vi "Data_Aquisition_cRIO7.vi"() -> ()   [LabVIEW 2016]
uses:
  <vilib>/Platform/TimedLoop/XDataNode/timing_clust.ctl
  <vilib>/Platform/TimedLoop/XDataNode/nitl_modes.ctl
  <vilib>/Platform/TimedLoop/XDataNode/wakeup.ctl
  <vilib>/Utility/file.llb/Write Delimited Spreadsheet (string).vi
  <vilib>/Platform/TimedLoop/XDataNode/loadnilvce.vi
  <vilib>/Utility/file.llb/Write Delimited Spreadsheet (DBL).vi
  <vilib>/Platform/TimedLoop/XDataNode/XDataNode.xnode
  <vilib>/Platform/TimedLoop/XDataNode/XDNodeRunTimeDep.lvlib
panel:
  in  "Mod 8 Labels":string[][](array[string])
  in  "Mod 6 Labels":string[][](array[string])
  in  "Mod 3 Labels":string[][](array[string])
  in  "Mod 2 Labels":string[][](array[string])
  in  "Mod 1 Labels":string[][](array[string])
  out "File Headers":string[][](array[string])=[["Unix Time Code", "M1AI0", "M1AI1", "M1AI2", "M1AI3", "M1AI4", "M1AI5", "M1AI6", "M1AI7", "M2DO0", "M2DO1", "M2DO3  ", "M2DO4", "M2DO4", "M2DO5", "M2DO6", "M2DO7", "M3AO0", "M3AO1", "M3AO2", "M3AO3", "M4DO0", "M4DO1", "M4DO2", "M4DO3", "M4DO4", "M4DO5", "M4DO6", "M4DO7", "M5AI0", "M5AI1", "M5AI2", "M5AI3", "M5AI4", "M5AI5", "M5AI6", "M5AI7", "M6AI0", "M6AI1", "M6AI2", "M6AI3", "M6AI4", "M6AI5", "M6AI6", "M6AI7", "M6AI16", "M6AI7", "M6AI18", "M6AI19", "M6AI20", "M6AI21", "M6AI22", "M6AI23", "M7DO0", "M7DO1", "M7DO3  ", "M7DO4", "M7DO4", "M7DO5", "M7DO6", "M7DO7", "M3AO0", "M3AO1", "M3AO2", "M3AO3"], ["Unix Time Code", "R1 pH", "N/A", "R1 N2  ", "N/A", "R1 Air", "R2 DO", "R2 Air", "R2 N2", "R1 Media Pump", "R1 Water Pump", "R1 Eff Pump", "R1 Gas Pump", "R1 Acid Pump", "R1 Base Pump", "R2 Air Valve", "R1 Release Valve", "R1 Air MFC", "R1 N2 MFC", "N/A", "N/A", "R2 Water Pump", "R2 Media Pump", "R2 Eff Pump", "R2 Acid Pump", "R2 Base Pump", "R2 Gas Pump", "R2 Release Valve", "R2 N2 Valve", "R2 pH", "N/A", "N/A", "N/A", "N/A", "N/A", "N/A", "N/A", "R1 DO ", "N/A", "R1 NH4+", "N/A", "R1 Ca2+", "N/A", "R1 K+", "N/A", "R1 Na+", "N/A", "R1 Cl-", "N/A", "R1 NO3-", "N/A", "R1 ORP", "N/A", "N/A", "N/A", "N/A", "R2 Water Pump 2", "R2 Floc FAir Valve", "R2 Floc Eff Pump", "R2 Floc Return Pump", "N/A", "R1 Air MFC", "R1 N2 MFC", "N/A", "N/A"]]
  in  "Buffer Size":i32=100
  out "Saving?":bool=TRUE
  out "new file path (Not A Path if cancelled)":path=path "u:/_03162018_194505.csv"
  in  "File Name:":string
  out "error out":errorcluster={"status"=TRUE, "code"=7, "source"="Open/Create/Replace File in Write Spreadsheet String.vi->Write Delimited Spreadsheet (string).vi->Data_Aquisition_cRIO1.vi<APPEND>\n/u/_03132018_011937.csv"}
  out "iter number":i32=109873
  in  "stop":bool
  out "All data":dbl[][](array[numeric]) format="%#3.4f"
  in  "error in":errorcluster
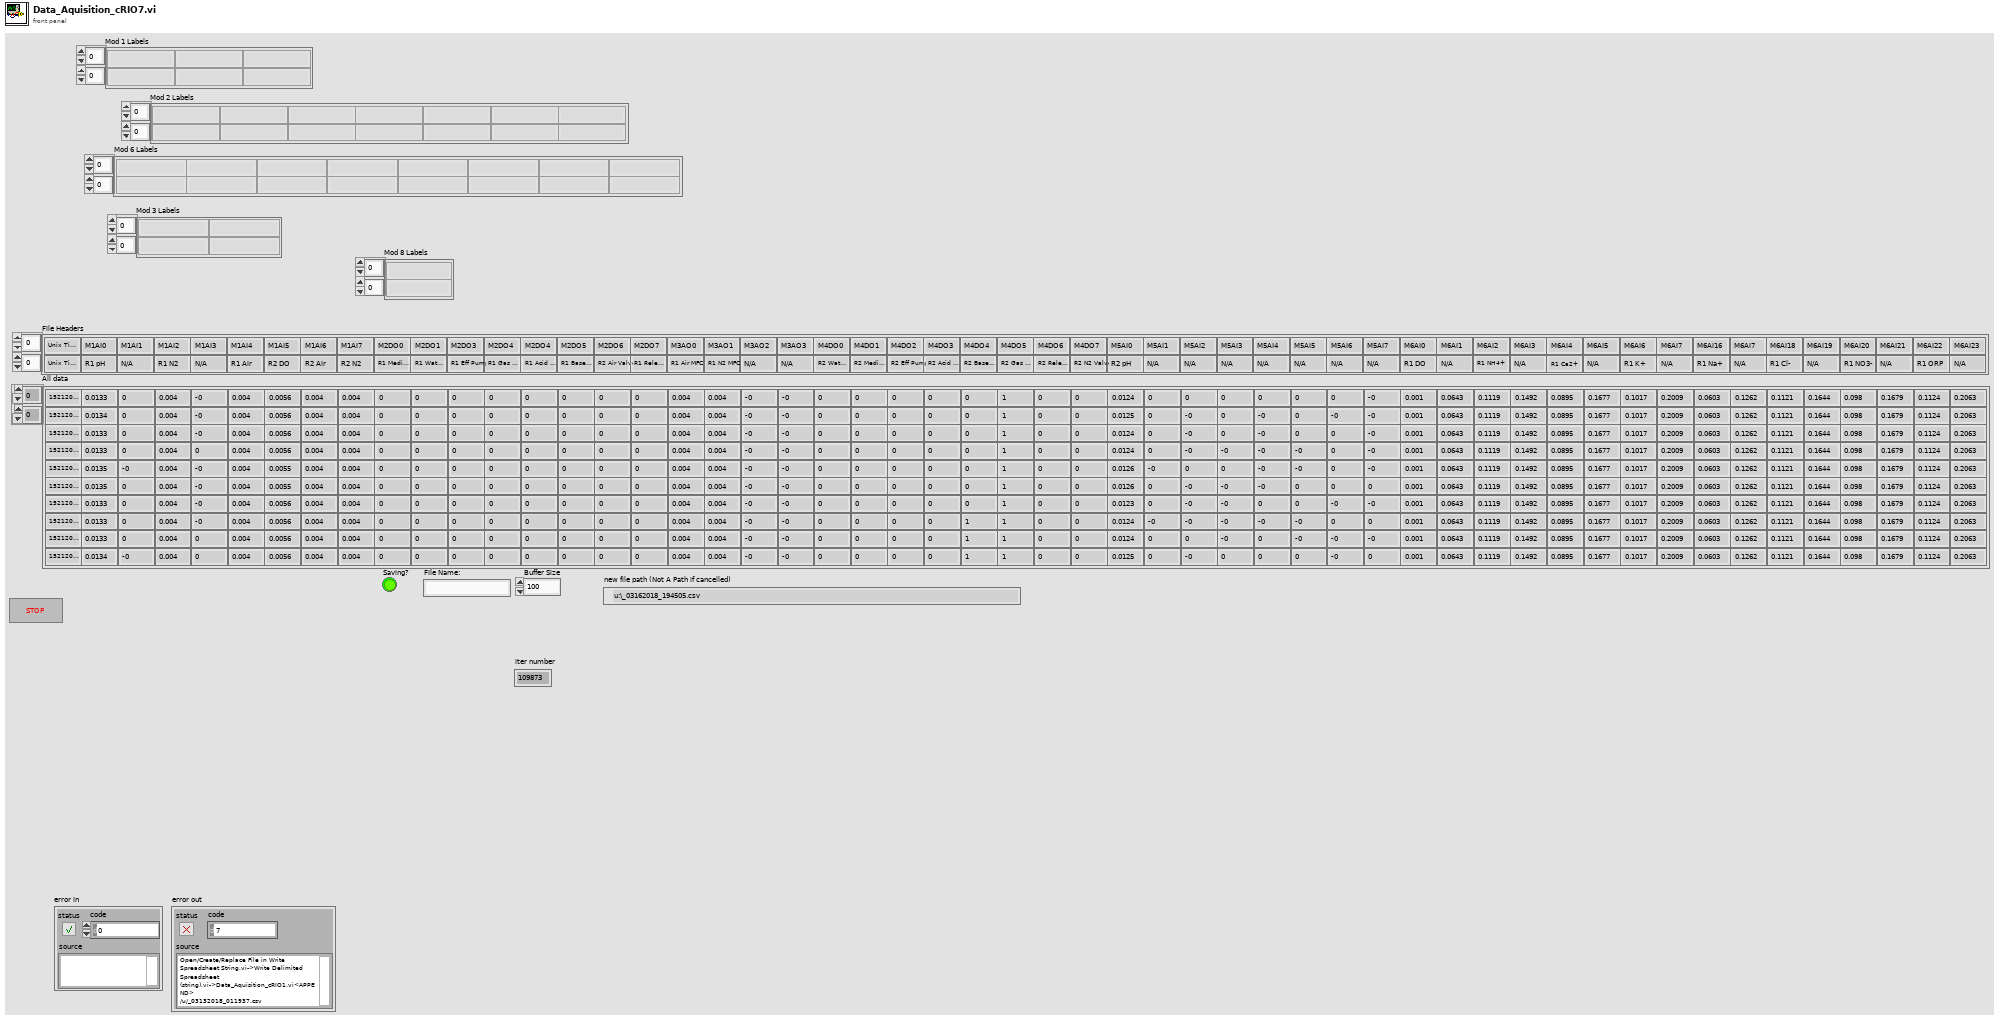
[diagram p1: front panel]
types:
  T1 = typedef "XDNodeRunTimeDep.lvlib/timing_clust.ctl" = cluster{"Expected End [f-1]":u64, "Actual End [f-1]":u64, "Finished Late? [f-1]":bool, "Expected End [i-1]":u64, "Actual End [i-1]":u64, "Finished Late? [i-1]":bool, "Expected Start [i]":u64, "Actual Start [i]":u64, "Expected Start [f]":u64, "Actual Start [f]":u64, "Source Name":string, "Structure Name":string, "Period":i64, "Deadline":i64, "Offset":i64, "Start":i64, "Priority":i32, "Timeout":i32, "Mode":T2, "Wakeup Reason":T3, "Error":errorcluster, "Source Type":string, "Secondary Source Type":string, "Global End Time":u64, "Global Start Time":u64, "Frame Duration":u64, "Iteration Duration":u64, "Assigned CPU":i32, "I/O Scan Engine Mode":u32}
  T2 = typedef "XDNodeRunTimeDep.lvlib/nitl_modes.ctl" = enum32{"No Change", "Process missed periods, maintain original phase", "Discard missed periods, maintain original phase", "Process missed periods, ignore original phase", "Discard missed periods, ignore original phase"}
  T3 = typedef "XDNodeRunTimeDep.lvlib/wakeup.ctl" = enum32{"Normal", "Aborted", "Asynchronous wakeup", "Timing source error", "Timed loop error", "Timeout"}
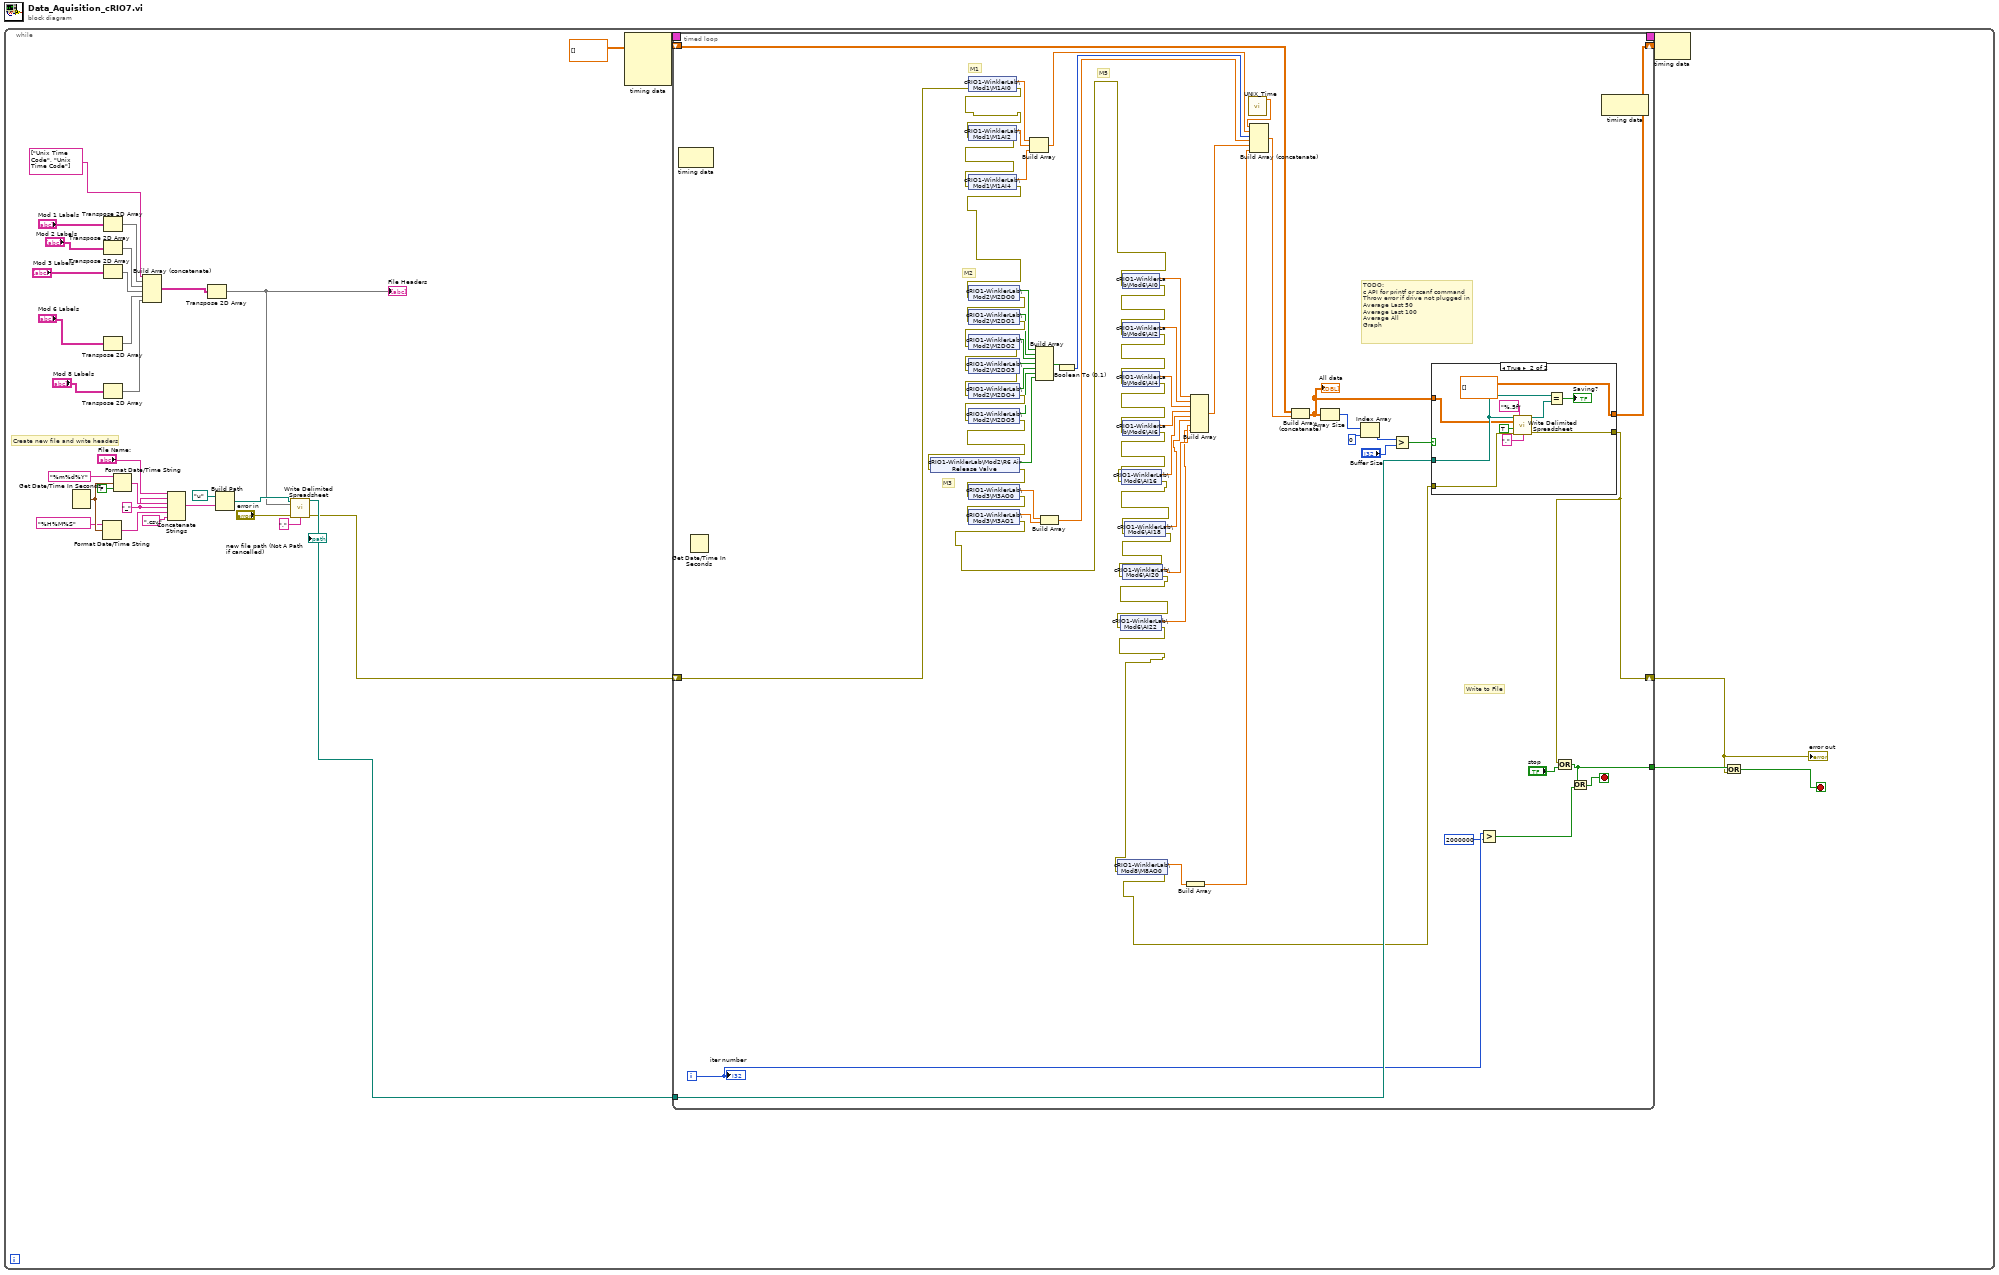
[diagram p0: block diagram]
diagram:
  n1 = while {
    stop <- w6 stop-if-true
    w23 = "_" ("string")
    # "Create new file and write headers"
    n2 = Get Date/Time In Seconds() -> (seconds since 1Jan1904=w28:timestamp)
    n3 = Format Date/Time String(time format string (%c)="%H%M%S", seconds (now)=w28) -> (date/time string=w22:string)  [unwired: 1 in]
    n4 = Transpose 2D Array(2D array="Mod 1 Labels") -> (transposed array=w15:string[][])
    n5 = Transpose 2D Array(2D array="Mod 2 Labels") -> (transposed array=w14:string[][])
    n6 = Transpose 2D Array(2D array="Mod 3 Labels") -> (transposed array=w13:string[][])
    n7 = Transpose 2D Array(2D array="Mod 6 Labels") -> (transposed array=w10:string[][])
    n8 = Transpose 2D Array(2D array="Mod 8 Labels") -> (transposed array=w9:string[][])
    n9 = Format Date/Time String(time format string (%c)="%m%d%Y", seconds (now)=w28, UTC format=FALSE) -> (date/time string=w24:string)
    n10 = Build Array (concatenate)(string[] ["Unix Time Code", "Unix Time Code"], w15, w14, w13, w10, w9) -> (w16:string[][])
    n11 = Concatenate Strings("File Name:", w23, w24, w23, w22, ".csv" ("string")) -> (w21:string)
    n12 = Transpose 2D Array(2D array=w16) -> (transposed array=w12:string[][])
    "File Headers" <- w12
    n13 = Build Path(base path=path "u:/" ("Save to:"), name or relative path=w21) -> (appended path=w31:path)
    n14 = call-poly <vilib>:"Write Delimited Spreadsheet.vi"("file path (dialog if empty)"=w31, "2D data"=w12, "error in (no error)"="error in", "delimiter (\\t)"="," ("delimiter (\\t)")) -> ("new file path (Not A Path if cancelled)"=w35:path, "error out"=w34:errorcluster)  [unwired: 10 in]
    "new file path (Not A Path if cancelled)" <- w35
    n15 = node-c288() -> (w20:T1)  [unwired: 4 in]
    n16 = timed-loop {
      tunnel: w35 -> [w97]
      shift-right: [w72] -> _
      shift-left: dbl[][] [] -> [w102]
      shift-right: [w66] -> w7
      shift-left: w34 -> [w70]
      tunnel: [w61] -> w8
      timing: w20 -> [_]
      timing-out: [_] -> w19
      i -> [w65]
      stop <- w62 stop-if-true
      # "M5"
      # "M3"
      # "M2"
      # "M1"
      # "TODO: \nc API for printf or scanf command\nThrow error if drive not plugged in\nAverage Last 50\nAverage Last 100\nAverage All\nGraph"
      # "Write to File"
      n17 = node-c288() -> ()  [unwired: 1 in, 1 out]
      n18 = Get Date/Time In Seconds() -> ()  [unwired: 1 out]
      n19 = shared-variable "cRIO1-WinklerLab\\Mod1\\M1AI0"(error in=w70) -> (w79:dbl, error out=w59:errorcluster)
      n20 = shared-variable "cRIO1-WinklerLab\\Mod1\\M1AI2"(error in=w59) -> (w56:dbl, error out=w58:errorcluster)
      n21 = shared-variable "cRIO1-WinklerLab\\Mod1\\M1AI4"(error in=w58) -> (w55:dbl, error out=w57:errorcluster)
      n22 = shared-variable "cRIO1-WinklerLab\\Mod2\\M2DO0"(error in=w57) -> (w80:bool, error out=w86:errorcluster)
      n23 = shared-variable "cRIO1-WinklerLab\\Mod2\\M2DO1"(error in=w86) -> (w81:bool, error out=w87:errorcluster)
      n24 = shared-variable "cRIO1-WinklerLab\\Mod2\\M2DO2"(error in=w87) -> (w82:bool, error out=w88:errorcluster)
      n25 = shared-variable "cRIO1-WinklerLab\\Mod2\\M2DO3"(error in=w88) -> (w83:bool, error out=w89:errorcluster)
      n26 = shared-variable "cRIO1-WinklerLab\\Mod2\\M2DO4"(error in=w89) -> (w84:bool, error out=w90:errorcluster)
      n27 = shared-variable "cRIO1-WinklerLab\\Mod2\\M2DO5"(error in=w90) -> (w85:bool, error out=w54:errorcluster)
      n28 = shared-variable "cRIO1-WinklerLab\\Mod2\\R6 Air Release Valve"(error in=w54) -> (w53:bool, error out=w94:errorcluster)
      n29 = shared-variable "cRIO1-WinklerLab\\Mod3\\M3AO0"(error in=w94) -> (w91:dbl, error out=w93:errorcluster)
      n30 = shared-variable "cRIO1-WinklerLab\\Mod3\\M3AO1"(error in=w93) -> (w92:dbl, error out=w52:errorcluster)
      n31 = Build Array(w79, w56, w55) -> (w78:dbl[])
      n32 = Build Array(w80, w81, w82, w83, w84, w85, w53) -> (w77:bool[])
      n33 = Build Array(w91, w92) -> (w75:dbl[])
      n34 = Boolean To (0,1)(Boolean=w77) -> (0, 1=w76:i16[])
      n35 = shared-variable "cRIO1-WinklerLab\\Mod6\\AI0"(error in=w52) -> (w95:dbl, error out=w51:errorcluster)
      n36 = shared-variable "cRIO1-WinklerLab\\Mod6\\AI2"(error in=w51) -> (w42:dbl, error out=w50:errorcluster)
      n37 = shared-variable "cRIO1-WinklerLab\\Mod6\\AI4"(error in=w50) -> (w41:dbl, error out=w49:errorcluster)
      n38 = shared-variable "cRIO1-WinklerLab\\Mod6\\AI6"(error in=w49) -> (w40:dbl, error out=w48:errorcluster)
      n39 = shared-variable "cRIO1-WinklerLab\\Mod6\\AI16"(error in=w48) -> (w39:dbl, error out=w47:errorcluster)
      n40 = shared-variable "cRIO1-WinklerLab\\Mod6\\AI18"(error in=w47) -> (w38:dbl, error out=w46:errorcluster)
      n41 = shared-variable "cRIO1-WinklerLab\\Mod6\\AI20"(error in=w46) -> (w37:dbl, error out=w45:errorcluster)
      n42 = shared-variable "cRIO1-WinklerLab\\Mod6\\AI22"(error in=w45) -> (w36:dbl, error out=w44:errorcluster)
      n43 = shared-variable "cRIO1-WinklerLab\\Mod8\\M8AO0"(error in=w44) -> (w74:dbl, error out=w43:errorcluster)
      n44 = Build Array(w74) -> (w67:dbl[])
      n45 = Build Array(w95, w42, w41, w40, w39, w38, w37, w36) -> (w68:dbl[])
      n46 = call "UNIX_Time.vi"() -> ("Unix time"=w69:dbl)  [unwired: 10 in, 1 out]
      n47 = Build Array (concatenate)(w69, w78, w76, w75, w68, w67) -> (w73:dbl[])
      n48 = Build Array (concatenate)(w102, w73) -> (w71:dbl[][])
      "All data" <- w71
      n49 = Array Size(array=w71) -> (size(s)=w101:i32[])
      n50 = Index Array(array=w101, index=0) -> (element=w99:i32)
      n51 = Greater?(x=w99, y="Buffer Size") -> (0:w98:bool)
      n52 = case shown="True" w98 {
        tunnel: w71 -> [w106 w107]
        tunnel: w97 -> [_ w114]
        tunnel: [w106 dbl[][] []] -> w72
        tunnel: [w105 w113] -> w66
        tunnel: w43 -> [w105 w108]
        frame False {
        }
        frame True {
          n53 = call-poly <vilib>:"Write Delimited Spreadsheet.vi"("file path (dialog if empty)"=w114, "format (%.3f)"="%.5f", "2D data"=w107, "append to file? (new file:F)"=TRUE, "error in (no error)"=w108, "delimiter (\\t)"="," ("delimiter (\\t)")) -> ("new file path (Not A Path if cancelled)"=w115:path, "error out"=w113:errorcluster)  [unwired: 8 in]
          n54 = Equal?(x=w114, y=w115) -> (x = y?=→"Saving?":bool)
        }
      }
      n55 = Greater?(x=w65, y=2000000) -> (0:w60:bool)
      n56 = Compound Arithmetic op=OR(w66, "stop") -> (w61:bool)
      n57 = Or(x=w61, y=w60) -> (x .or. y?=w62:bool)
      n58 = node-c288() -> ()  [unwired: 1 in, 1 out]
      "iter number" <- w65
    }
    "error out" <- w7
    n59 = node-c288(w19) -> ()  [unwired: 1 out]
    n60 = Or(x=w8, y=w7) -> (x .or. y?=w6:bool)
  }
